vi "Calling VI Ref If Not Valid.vi"(4 "Chain Index":i32=-1, 6 "Open Relationship (Caller)":T1(ring)=enum."Calling VI", 8 "error in (no error)":errorcluster, 9 "VI Reference":refnum<vi>) -> (0 "error out":errorcluster, 1 "Valid VI Ref":refnum<vi>, 2 "New Reference Opened":bool)   [LabVIEW 2023]
doc: "This VI will make a <B>Valid VI Ref</B> if the <B>VI Reference</B> being passed in is not valid. It does this by opening a reference to a VI in the chain. By default the calling VI will be opened but this can be changed with the enum <B>Open Relationship (Caller)</B> or the <B>Chain Index</B> controls.\n-------------\nBrian Hoover (hooovahh)"
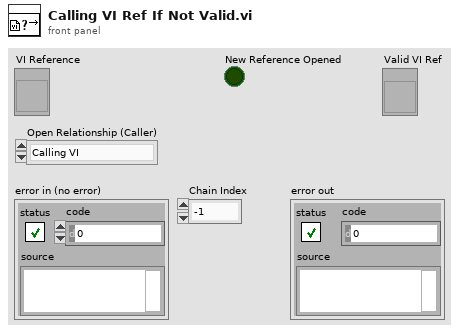
[diagram p1: front panel]
types:
  T1 = enum16{"This VI", "Calling VI", "Callers Caller", "Callers Callers Caller"}
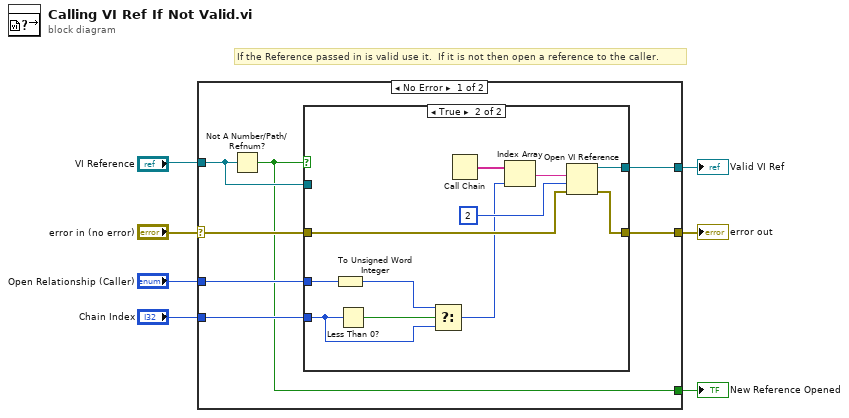
[diagram p0: block diagram]
diagram:
  # "If the Reference passed in is valid use it.  If it is not then open a reference to the caller."
  n1 = case shown="No Error" "error in (no error)" {
    selector: "error in (no error)" -> [w9 w29]
    tunnel: "VI Reference" -> [w14 w28]
    tunnel: [w13 w28] -> w6
    tunnel: [w12 w29] -> w5
    tunnel: "Open Relationship (Caller)" -> [w11 _]
    tunnel: "Chain Index" -> [w10 _]
    tunnel: [w8 _] -> w1
    frame No Error {
      n2 = Not A Number/Path/Refnum?(number/path/refnum=w14) -> (NaN/Path/Refnum?=w8:bool)
      n3 = case shown="True" w8 {
        tunnel: w14 -> [w16 _]
        tunnel: [w16 w24] -> w13
        tunnel: w9 -> [w15 w23]
        tunnel: [w15 w22] -> w12
        tunnel: w11 -> [_ w19]
        tunnel: w10 -> [_ w20]
        frame False {
        }
        frame True {
          n4 = To Unsigned Word Integer(number=w19) -> (unsigned 16bit integer=w17:u16)
          n5 = Less Than 0?(x=w20) -> (x < 0?=w21:bool)
          n6 = Select(t=w17, s=w21, f=w20) -> (s? t:f=w18:i32)
          n7 = Call Chain() -> (call chain=w27:string[])
          n8 = Index Array(array=w27, index=w18) -> (element=w26:string)
          n9 = Open VI Reference(vi path=w26, options=2, error in (no error)=w23) -> (vi reference=w24:refnum<vi>, error out=w22:errorcluster)  [unwired: 3 in]
        }
      }
    }
    frame Error {
    }
  }
  "Valid VI Ref" <- w6
  "error out" <- w5
  "New Reference Opened" <- w1
